vi "replaceValuesToken.vi"(8 "error in (no error)":errorcluster, 10 "Query":string, 11 "TransactionList in":refnum<class "TransactionList.lvclass">) -> (0 "error out":errorcluster, 2 "Query":string, 3 "TransactionList out":refnum<class "TransactionList.lvclass">)   [LabVIEW 2018, in "TransactionList.lvclass"]
uses:
  TransactionList.lvclass
  TransactionList.lvclass/TransactionList.ctl
  Transaction/Transaction.lvclass
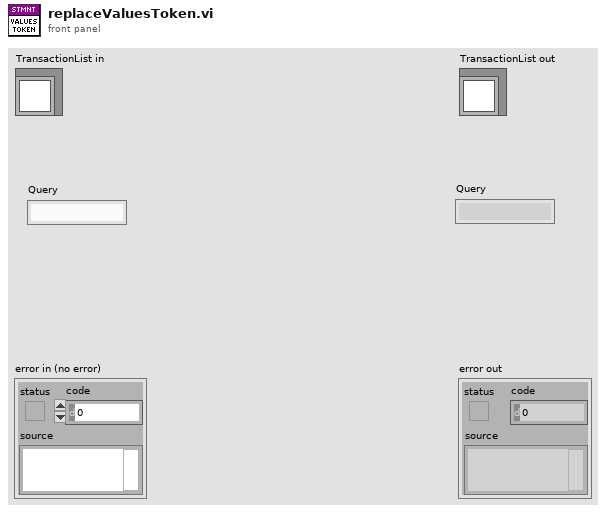
[diagram p1: front panel]
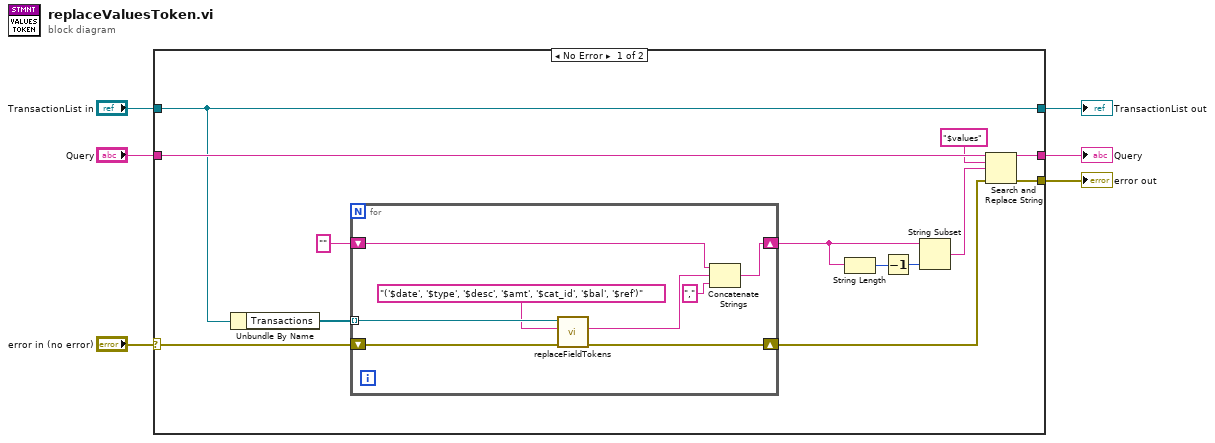
[diagram p0: block diagram]
diagram:
  n1 = case shown="No Error" "error in (no error)" {
    selector: "error in (no error)" -> [w13 w30]
    tunnel: [w19 w30] -> w5
    tunnel: [w16 w29] -> w3
    tunnel: "TransactionList in" -> [w16 w29]
    tunnel: [w18 w28] -> w2
    tunnel: "Query" -> [w17 w28]
    frame No Error {
      n2 = Unbundle By Name(w16) -> ("Transactions"=w15:refnum<class "Transaction.lvclass">[])
      n3 = for {
        tunnel: w15 -> [w24] mode=indexing
        shift-right: [w25] -> w10
        shift-left: "" -> [w26]
        shift-right: [w20] -> w8
        shift-left: w13 -> [w22]
        n4 = call-dynamic "replaceFieldTokens.vi"("error in (no error)"=w22, "Query In"="('$date', '$type', '$desc', '$amt', '$cat_id', '$bal', '$ref')", "Transaction in"=w24) -> ("error out"=w20:errorcluster, "Query Out"=w21:string)  [unwired: 6 in, 1 out]
        n5 = Concatenate Strings(w26, w21, "," ("string")) -> (w25:string)
      }
      n6 = String Length(string=w10) -> (length=w11:i32)
      n7 = Decrement(x=w11) -> (x-1=w12:i32)
      n8 = String Subset(string=w10, length (rest)=w12) -> (substring=w9:string)  [unwired: 1 in]
      n9 = Search and Replace String(input string=w17, search string="$values", replace string=w9, error in=w8) -> (result string=w18:string, error out=w19:errorcluster)  [unwired: 4 in, 2 out]
    }
    frame Error {
    }
  }
  "error out" <- w5
  "TransactionList out" <- w3
  "Query" <- w2
